vi "写文本转字符协议.vi"(10 "输入文本":string, 11 "输入地址":i32) -> (2 "返回字节数":u16, 3 "连接的字符串":string)   [LabVIEW 2012]
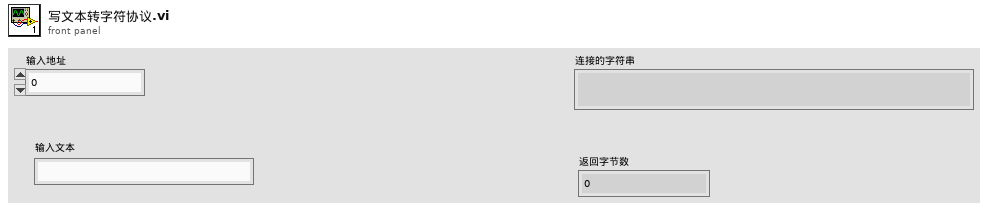
[diagram p1: front panel]
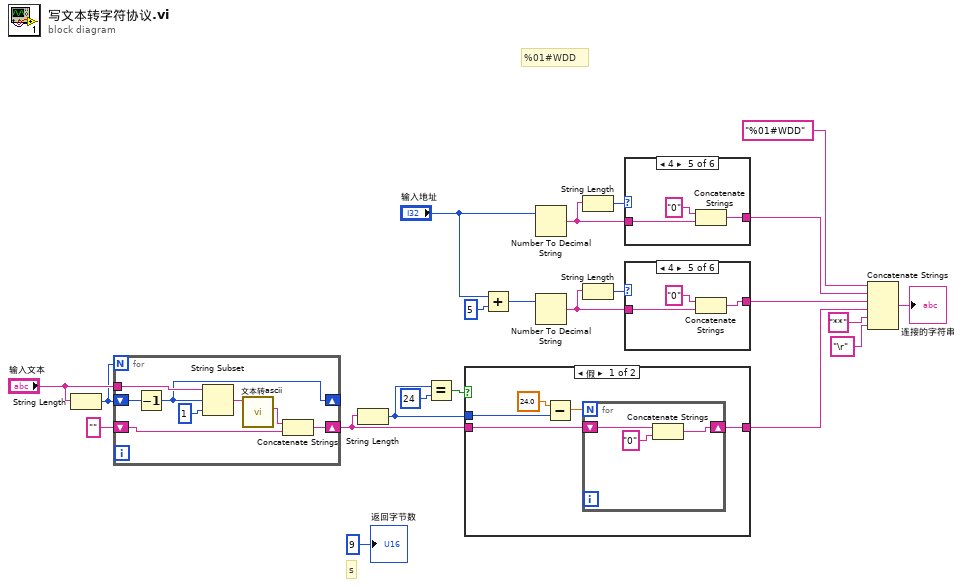
[diagram p0: block diagram]
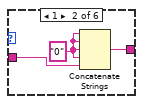
[diagram p4: hidden frame]
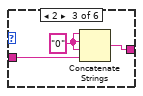
[diagram p5: hidden frame]
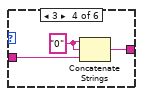
[diagram p6: hidden frame]
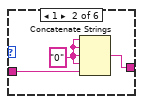
[diagram p9: hidden frame]
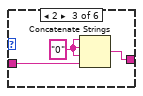
[diagram p10: hidden frame]
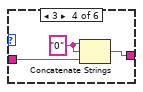
[diagram p11: hidden frame]
diagram:
  # "s"
  # "%01#WDD"
  n1 = String Length(string="输入文本") -> (length=w7:i32)
  n2 = for {
    N: w7 -> [_]
    tunnel: "输入文本" -> [w30]
    shift-right: [w25] -> _
    shift-left: w7 -> [w26]
    shift-right: [w27] -> w3
    shift-left: "" -> [w28]
    n3 = Decrement(x=w26) -> (x-1=w25:i32)
    n4 = String Subset(string=w30, offset (0)=w25, length (rest)=1 ("长度（剩余）")) -> (substring=w24:string)
    n5 = call "文本转ascii.vi"("文本输入"=w24) -> ("字符串"=w23:string)  [unwired: 9 in, 1 out]
    n6 = Concatenate Strings(w23, w28) -> (w27:string)
  }
  n7 = String Length(string=w3) -> (length=w2:i32)
  n8 = Equal?(x=w2, y=24) -> (x = y?=w4:bool)
  n9 = case shown="假" w4 {
    tunnel: [w34 w39] -> w1
    tunnel: w3 -> [w35 w39]
    tunnel: w2 -> [w32 _]
    frame False {
      n10 = Subtract(x=24.0, y=w32) -> (x-y=w31:dbl)
      n11 = for {
        N: w31 -> [_]
        shift-right: [w36] -> w34
        shift-left: w35 -> [w38]
        n12 = Concatenate Strings(w38, "0" ("字符串")) -> (w36:string)
      }
    }
    frame True {
    }
  }
  n13 = Add(x="输入地址", y=5) -> (x+y=w10:i32)
  n14 = Number To Decimal String(number="输入地址") -> (decimal integer string=w13:string)  [unwired: 1 in]
  n15 = Number To Decimal String(number=w10) -> (decimal integer string=w9:string)  [unwired: 1 in]
  n16 = String Length(string=w13) -> (length=w21:i32)
  n17 = String Length(string=w9) -> (length=w14:i32)
  n18 = case shown="4" w21 {
    tunnel: w13 -> [w40 w43 w46 w49 w52 w53]
    tunnel: [w40 w41 w44 w47 w50 w53] -> w20
    frame 0, Default {
    }
    frame 1 {
      w42 = "0" ("字符串")
      n19 = Concatenate Strings(w42, w42, w42, w42, w43) -> (w41:string)
    }
    frame 2 {
      w45 = "0" ("字符串")
      n20 = Concatenate Strings(w45, w45, w45, w46) -> (w44:string)
    }
    frame 3 {
      w48 = "0" ("字符串")
      n21 = Concatenate Strings(w48, w48, w49) -> (w47:string)
    }
    frame 4 {
      n22 = Concatenate Strings("0" ("字符串"), w52) -> (w50:string)
    }
    frame 5 {
    }
  }
  n23 = case shown="4" w14 {
    tunnel: w9 -> [_ w56 w59 w62 w65 w66]
    tunnel: [_ w54 w57 w60 w63 w66] -> w15
    frame 0, Default {
    }
    frame 1 {
      w55 = "0" ("字符串")
      n24 = Concatenate Strings(w55, w55, w55, w55, w56) -> (w54:string)
    }
    frame 2 {
      w58 = "0" ("字符串")
      n25 = Concatenate Strings(w58, w58, w58, w59) -> (w57:string)
    }
    frame 3 {
      w61 = "0" ("字符串")
      n26 = Concatenate Strings(w61, w61, w62) -> (w60:string)
    }
    frame 4 {
      n27 = Concatenate Strings("0" ("字符串"), w65) -> (w63:string)
    }
    frame 5 {
    }
  }
  n28 = Concatenate Strings("%01#WDD" ("字符串"), w20, w15, w1, "**" ("字符串"), "\r" ("字符串")) -> (→"连接的字符串":string)
  "返回字节数" <- u16 9 ("返回字节数")
